vi "Database_Main_V1.0.0-a.2.vi"() -> ()   [LabVIEW 2020]
uses:
  <vilib>/addons/database/Connection.llb/DB Tools Open Connec (String).vi
  <vilib>/addons/database/Connection.llb/Conn Execute.vi
  <vilib>/addons/database/Recordset.llb/Rec Destroy - Connection.vi
  <vilib>/addons/database/_DB Variant To Data/Database Variant To Data.xnode
  <vilib>/addons/database/NI_Database_API.lvlib
panel:
  out "Table Control":string[][](table)
  out "Resulting SQL Query":string
  in  "Table name":string="Data"
  in  "Project_ID":string="Value"
  in  "Delete":bool
  in  "Printing_Date":string
  in  "Modell_Name":string
  in  "Printer_Type":string
  in  "Project_Status":string
  in  "Results 2":dbl format="%#_13g"
  in  "Results":i32
  in  "Project_ID":string="ProjectX"
  in  "Write":bool
  in  "stop":bool
  in  "Read":bool
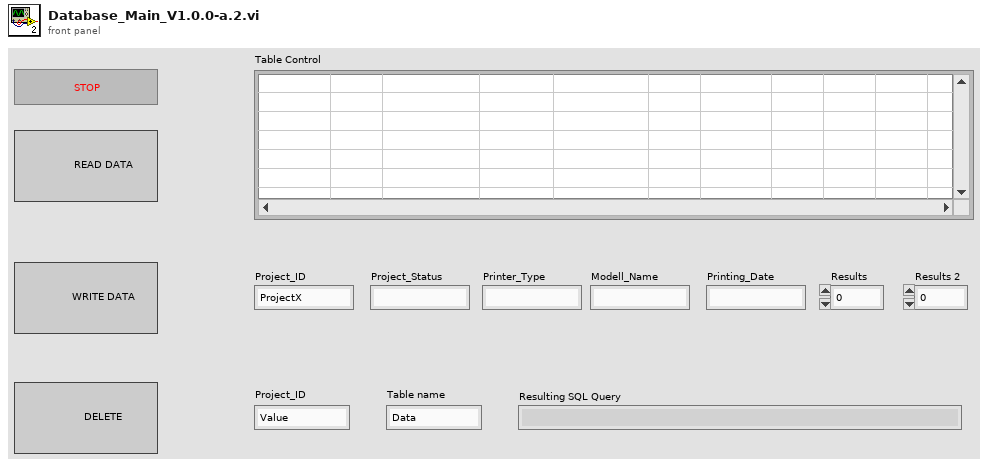
[diagram p1: front panel]
types:
  T1 = cluster{string, string, string, string, string, i32, dbl}[]
  T2 = typedef "NI_Database_API.lvlib/Conn ObjectReference.ctl" = refnum<k1>
  T3 = cluster{"Project_ID":string, "Project_Status":string, "Printer_Type":string, "Modell_Name":string, "Printing_Date":string, "Results":i32, "Results 2":dbl}
  T4 = typedef "NI_Database_API.lvlib/Rec ObjectReference.ctl" = refnum<k1>
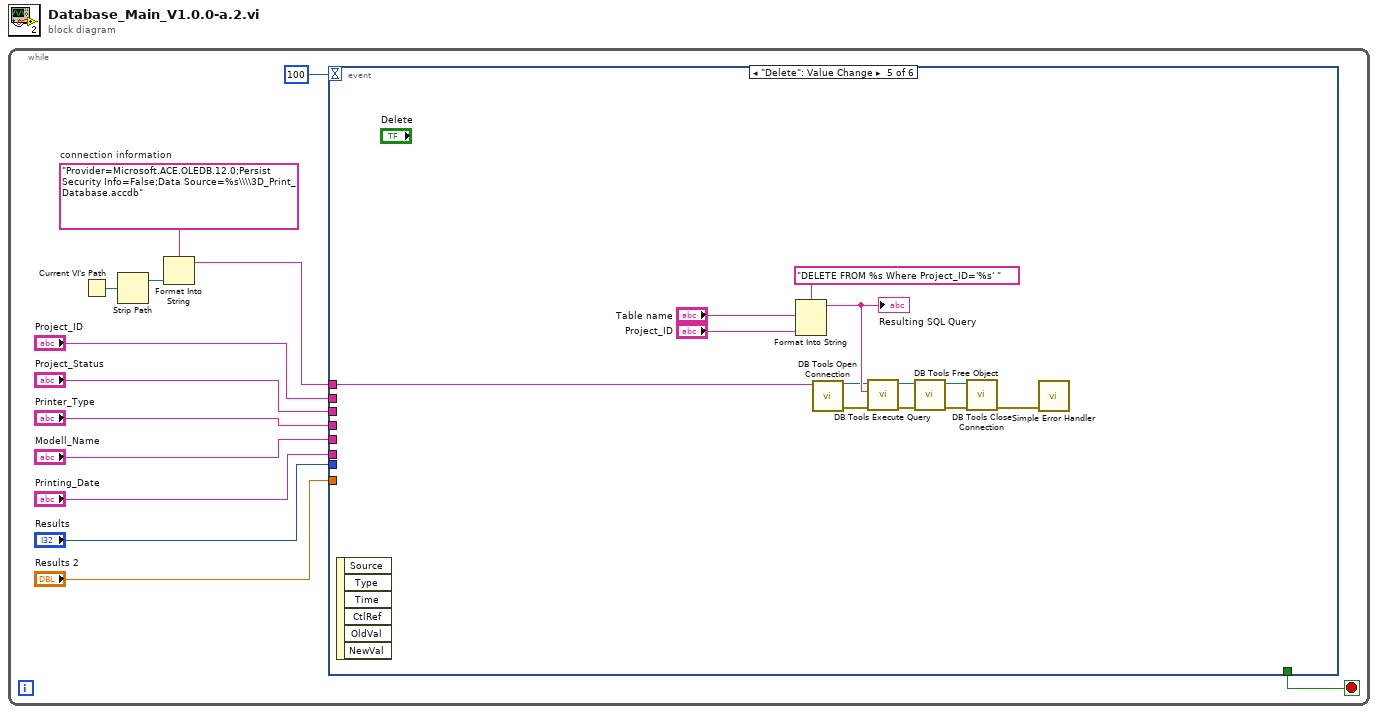
[diagram p0: block diagram]
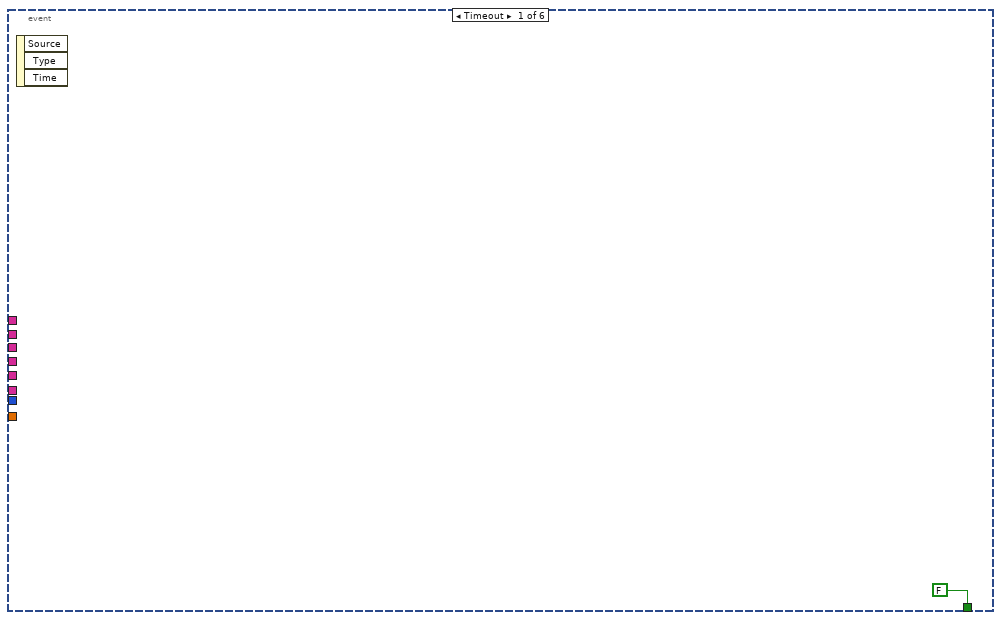
[diagram p2: hidden frame]
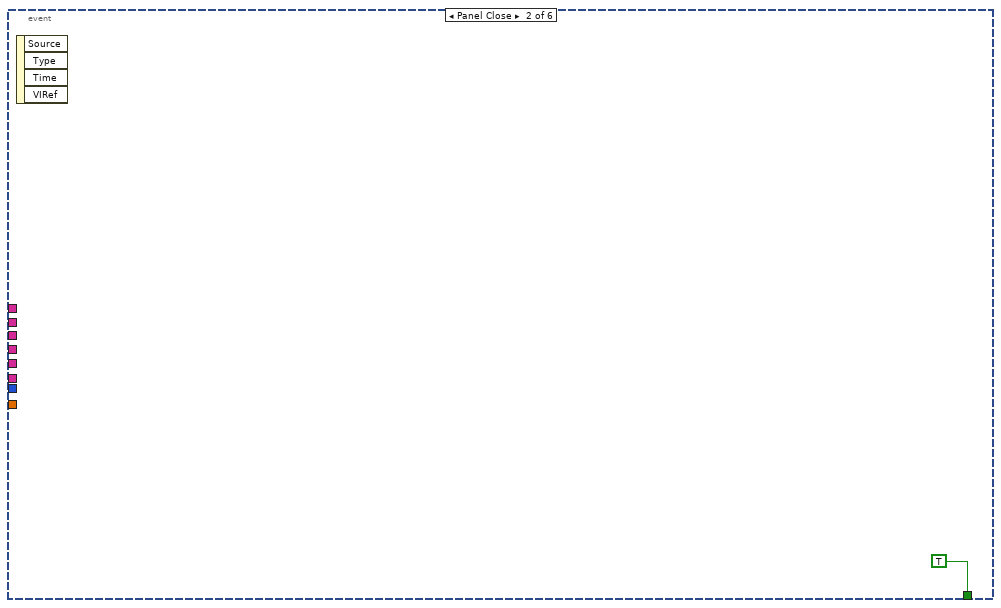
[diagram p3: hidden frame]
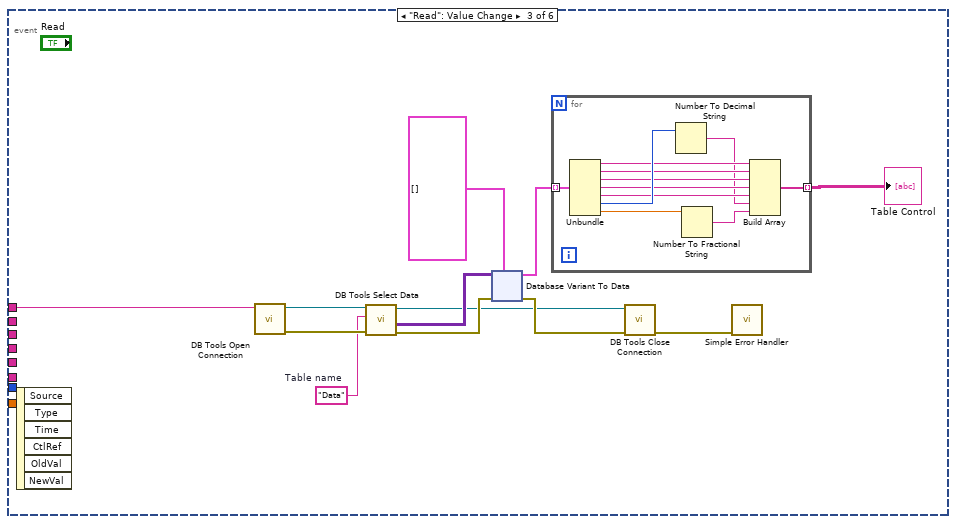
[diagram p4: hidden frame]
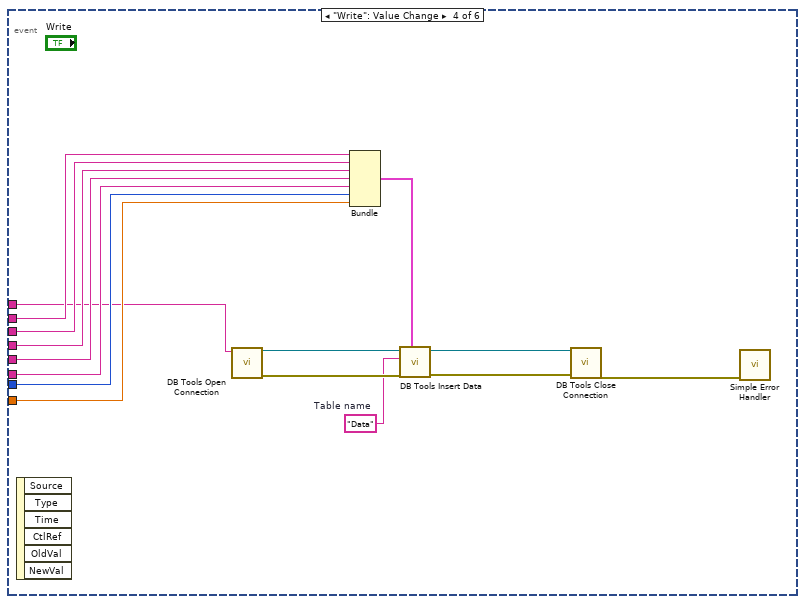
[diagram p5: hidden frame]
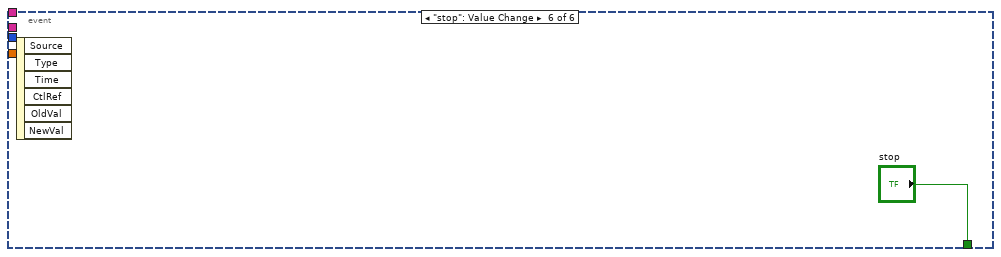
[diagram p6: hidden frame]
diagram:
  n1 = while {
    stop <- w13 stop-if-true
    w10 = "Provider=Microsoft.ACE.OLEDB.12.0;Persist Security Info=False;Data Source=%s\\\\3D_Print_Database.accdb"  # connection information
    n2 = Current VI's Path() -> (path=w9:path)
    n3 = Strip Path(path=w9) -> (stripped path=w11:path)  [unwired: 1 out]
    n4 = Format Into String(format string=w10, w11) -> (resulting string=w8:string)  [unwired: 2 in, 1 out]
    n5 = event shown="[4] \"Delete\": Value Change" {
      selector: _ -> [_ _ _ _ _ _]
      dyn-events: _ -> [_ _ _ _ _ _]
      timeout: 100 -> [_ _ _ _ _ _]
      tunnel: [FALSE TRUE _ _ _ "stop"] -> w13
      tunnel: w8 -> [_ _ w17 w266 w282 _]
      tunnel: "Project_ID" -> [_ _ _ w273 _ _]
      tunnel: "Project_Status" -> [_ _ _ w272 _ _]
      tunnel: "Printer_Type" -> [_ _ _ w271 _ _]
      tunnel: "Modell_Name" -> [_ _ _ w270 _ _]
      tunnel: "Printing_Date" -> [_ _ _ w269 _ _]
      tunnel: "Results" -> [_ _ _ w268 _ _]
      tunnel: "Results 2" -> [_ _ _ w267 _ _]
      event Timeout {
        n6 = event-data() -> ()  [unwired: 1 in, 3 out]
      }
      event Panel Close {
        n7 = event-data() -> ()  [unwired: 1 in, 4 out]
      }
      event "Read": Value Change {
        w18 = "Data"  # Table name
        n8 = event-data() -> ()  [unwired: 1 in, 6 out]
        n9 = call-poly <vilib>:"DB Tools Open Connection.vi"("connection information"=w17) -> ("error out"=w26:errorcluster, "connection reference"=w27:T2)  [unwired: 7 in]
        n10 = call <vilib>:"DB Tools Select Data.vi"("error in (no error)"=w26, "table"=w18, "connection reference"=w27) -> ("error out"=w25:errorcluster, "data"=w24:variant[][], "connection reference out"=w19:T2)  [unwired: 3 in]
        n11 = xnode "Database Variant To Data"("database variant"=w24, "error in (no error)"=w25, "type"=T1 []) -> ("data"=w21:T1, "error out"=w20:errorcluster)
        n12 = for {
          tunnel: w21 -> [w38] mode=indexing
          tunnel: [w34] -> w16 mode=indexing
          n13 = Unbundle "Unbundle"(w38) -> (w36:string, w35:string, w33:string, w32:string, w31:string, w37:i32, w29:dbl)
          n14 = Number To Decimal String(number=w37) -> (decimal integer string=w30:string)  [unwired: 1 in]
          n15 = Number To Fractional String(number=w29) -> (F-format string=w28:string)  [unwired: 3 in]
          n16 = Build Array(w36, w35, w33, w32, w31, w30, w28) -> (w34:string[])
        }
        "Table Control" <- w16
        n17 = call <vilib>:"DB Tools Close Connection.vi"("error in (no error)"=w20, "connection reference"=w19) -> ("error out"=w23:errorcluster)  [unwired: 5 in]
        n18 = call <vilib>:"Simple Error Handler.vi"("error in (no error)"=w23) -> ()  [unwired: 4 in, 5 out]
      }
      event "Write": Value Change {
        w278 = "Data"  # Table name
        n19 = event-data() -> ()  [unwired: 1 in, 6 out]
        n20 = call-poly <vilib>:"DB Tools Open Connection.vi"("connection information"=w266) -> ("error out"=w279:errorcluster, "connection reference"=w280:T2)  [unwired: 7 in]
        n21 = Bundle "Bundle"("Project_ID"=w273, "Project_Status"=w272, "Printer_Type"=w271, "Modell_Name"=w270, "Printing_Date"=w269, "Results"=w268, "Results 2"=w267) -> (w277:T3)  [unwired: 1 in]
        n22 = call <vilib>:"DB Tools Insert Data.vi"("data"=w277, "error in (no error)"=w279, "table"=w278, "connection reference"=w280) -> ("error out"=w275:errorcluster, "connection reference out"=w276:T2)  [unwired: 6 in]
        n23 = call <vilib>:"DB Tools Close Connection.vi"("error in (no error)"=w275, "connection reference"=w276) -> ("error out"=w274:errorcluster)  [unwired: 5 in]
        n24 = call <vilib>:"Simple Error Handler.vi"("error in (no error)"=w274) -> ()  [unwired: 4 in, 5 out]
      }
      event "Delete": Value Change {
        n25 = event-data() -> ()  [unwired: 1 in, 6 out]
        n26 = Format Into String(format string="DELETE FROM %s Where Project_ID='%s' ", "Table name", "Project_ID") -> (resulting string=w287:string)  [unwired: 2 in, 1 out]
        "Resulting SQL Query" <- w287
        n27 = call-poly <vilib>:"DB Tools Open Connection.vi"("connection information"=w282) -> ("error out"=w284:errorcluster, "connection reference"=w283:T2)  [unwired: 7 in]
        n28 = call-poly <vilib>:"DB Tools Execute Query.vi"("error in (no error)"=w284, "SQL query"=w287, "connection reference"=w283) -> ("error out"=w292:errorcluster, "recordset reference"=w291:T4)  [unwired: 5 in]
        n29 = call-poly <vilib>:"DB Tools Free Object.vi"("error in (no error)"=w292, "recordset reference"=w291) -> ("error out"=w290:errorcluster, "connection reference"=w289:T2)  [unwired: 8 in]
        n30 = call <vilib>:"DB Tools Close Connection.vi"("error in (no error)"=w290, "connection reference"=w289) -> ("error out"=w281:errorcluster)  [unwired: 5 in]
        n31 = call <vilib>:"Simple Error Handler.vi"("error in (no error)"=w281) -> ()  [unwired: 4 in, 5 out]
      }
      event "stop": Value Change {
        n32 = event-data() -> ()  [unwired: 1 in, 6 out]
      }
    }
  }
